vi "set range.vi"(8 "error in (no error)":errorcluster, 10 "Range (0: 1 - Lowest)":u16(ring) items=["1 - Lowest", "2", "3", "4", "5 - Highest"], 11 "VISA session":refnum<visa-resource-name>) -> (0 "error out":errorcluster, 3 "dup VISA session":refnum<visa-resource-name>)   [LabVIEW 2017]
panel:
  # "When you set this, it also turns autorange off, if it was on"
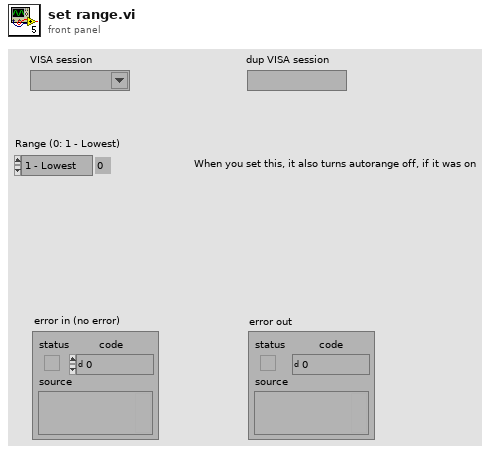
[diagram p1: front panel]
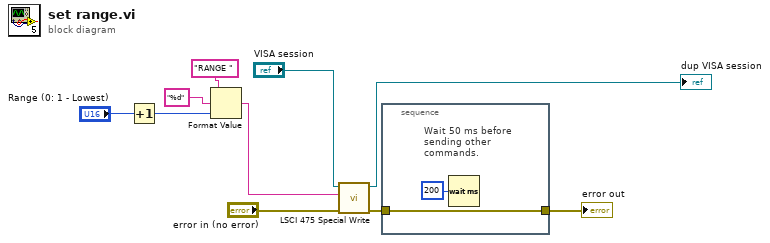
[diagram p0: block diagram]
diagram:
  n1 = Increment(x="Range (0: 1 - Lowest)") -> (x+1=w2:u16)
  n2 = Format Value(string ("")="RANGE ", format string="%d", value (0)=w2) -> (output string=w1:string)
  n3 = call "LSCI 475 Special Write.vi"("error in (no error)"="error in (no error)", "Write Buffer (\"\")"=w1, "VISA session"="VISA session") -> ("error out"=w7:errorcluster, "dup VISA session"=→"dup VISA session":refnum<visa-resource-name>)  [unwired: 6 in, 1 out]
  n4 = stacked-sequence {
    tunnel: w7 -> [w11]
    tunnel: [w11] -> w8
    frame #0 {
      # "Wait 50 ms before\nsending other\ncommands."
      n5 = Wait (ms)(milliseconds to wait=u32 200) -> ()  [unwired: 1 out]
    }
  }
  "error out" <- w8
